vi "INIScoreFile Add Score.vi"(8 "error in (no error)":errorcluster, 9 "Score":u32, 10 "Name":string, 11 "INIScoreFile in":refnum<class "INIScoreFile.lvclass">) -> (0 "error out":errorcluster, 3 "INIScoreFile out":refnum<class "INIScoreFile.lvclass">)   [LabVIEW 2020, in "INIScoreFile.lvclass"]
uses:
  INIScoreFile.lvclass
  INIScoreFile.lvclass/INIScoreFile.ctl
  9dfe2a9f-7995-457b-976a-632512e74ae6.vi
  9dfe2a9f-7995-457b-976a-632512e74ae6.vi/c0db33a9-eb6c-44d9-b982-8563e05d2734.vi
  9dfe2a9f-7995-457b-976a-632512e74ae6.vi/ae3535a8-0066-4e8d-a5de-b07ac05a7c65.vi
  9dfe2a9f-7995-457b-976a-632512e74ae6.vi/dda8e586-731b-4197-ad83-6a4d05585a0a.vi
  <vilib>/Comparison/Less/Less Functor/Less Functor.lvclass
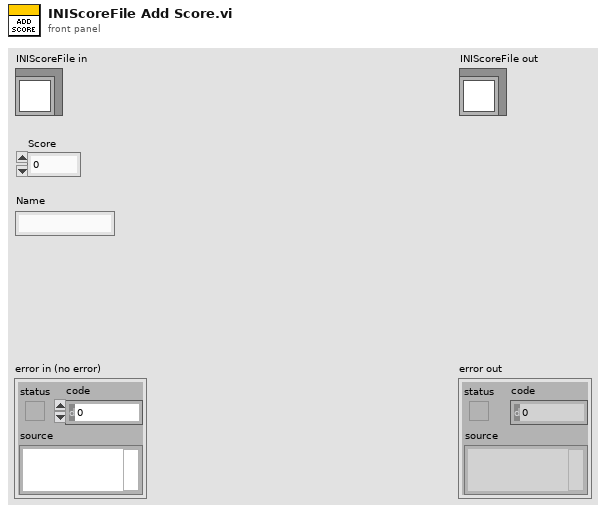
[diagram p1: front panel]
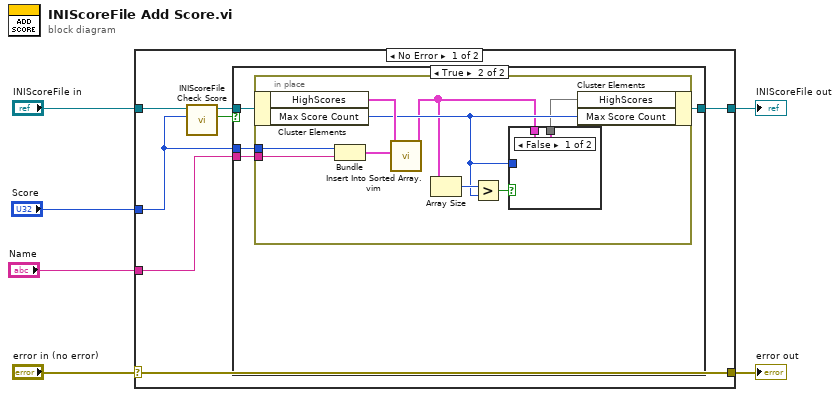
[diagram p0: block diagram]
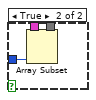
[diagram p3: hidden frame]
diagram:
  n1 = case shown="No Error" "error in (no error)" {
    selector: "error in (no error)" -> [w13 w33]
    tunnel: [w13 w33] -> w5
    tunnel: [w9 w32] -> w3
    tunnel: "INIScoreFile in" -> [w12 w32]
    tunnel: "Score" -> [w8 _]
    tunnel: "Name" -> [w7 _]
    frame No Error {
      n2 = call-dynamic "INIScoreFile Check Score.vi"("Score"=w8, "INIScoreFile in"=w12) -> ("Is High?"=w10:bool, "INIScoreFile out"=w11:refnum<class "INIScoreFile.lvclass">)  [unwired: 7 in, 1 out]
      n3 = case shown="True" w10 {
        tunnel: w11 -> [w14 w18]
        tunnel: [w14 w17] -> w9
        tunnel: w8 -> [_ w16]
        tunnel: w7 -> [_ w15]
        frame False {
        }
        frame True {
          n4 = in-place {
            in-place-border: w16 -> [w26]
            in-place-border: w15 -> [w25]
            n5 = in-place-cluster #1(w18) -> ("HighScores"=w27:cluster{"Score":u32, "Name":string}[], "Max Score Count"=w22:i32)
            n6 = Bundle("Score"=w26, "Name"=w25) -> (w24:cluster{"Score":u32, "Name":string})  [unwired: 1 in]
            n7 = call "Insert Into Sorted Array.vim"("element"=w24, "sorted array in"=w27) -> ("sorted array out"=w21:cluster{"Score":u32, "Name":string}[])  [unwired: 9 in]
            n8 = Array Size(array=w21) -> (size(s)=w23:i32)
            n9 = Greater?(x=w23, y=w22) -> (0:w19:bool)
            n10 = case shown="False" w19 {
              tunnel: w22 -> [_ w31]
              tunnel: w21 -> [w28 w30]
              tunnel: [w28 w29] -> w20
              frame False {
              }
              frame True {
                n11 = Array Subset(array=w30, length=w31) -> (w29:cluster{"Score":u32, "Name":string}[])  [unwired: 1 in]
              }
            }
            n12 = in-place-cluster #1("HighScores"=w20, "Max Score Count"=w22) -> (w17:refnum<class "INIScoreFile.lvclass">)
          }
        }
      }
    }
    frame Error {
    }
  }
  "error out" <- w5
  "INIScoreFile out" <- w3
